vi "acquireValue.vi"(8 "error in (no error)":errorcluster, 10 "nextSample?":bool, 11 "appliedSettingsMatchStart in":refnum<class "appliedSettingsMatchStart.lvclass">) -> (0 "error out":errorcluster, 1 "function return":i32, 2 "variantData":variant, 3 "appliedSettingsMatchStart out":refnum<class "appliedSettingsMatchStart.lvclass">)   [LabVIEW 2016, in "SALLV_AtDome_Messaging.lvlib" / "appliedSettingsMatchStart.lvclass"]
uses:
  appliedSettingsMatchStart.lvclass
  appliedSettingsMatchStart.lvclass/appliedSettingsMatchStart.ctl
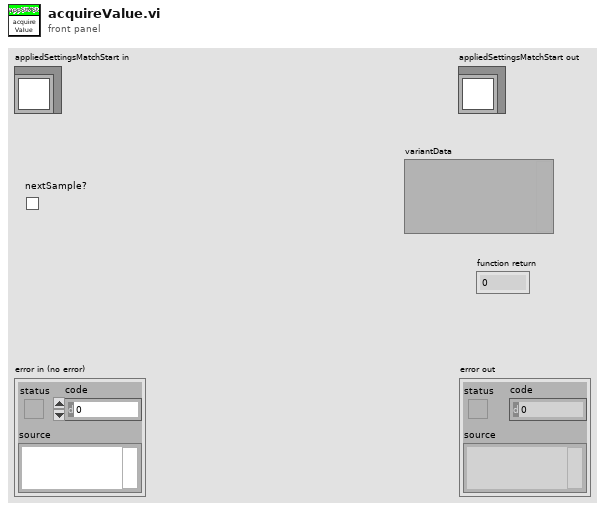
[diagram p1: front panel]
types:
  T1 = typedef "SALLV_EXA.lvlib/logevent_appliedSettingsMatchStart.ctl" = cluster{"appliedSettingsMatchStartIsTrue":bool, "priority":i32}
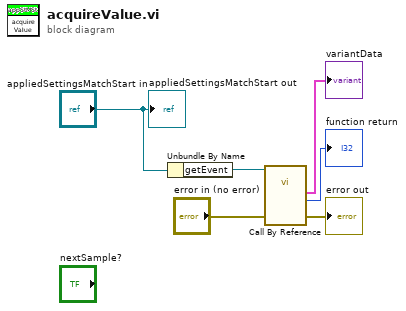
[diagram p0: block diagram]
diagram:
  n1 = Unbundle By Name("appliedSettingsMatchStart in") -> ("getEvent"=w6:refnum<vi>)
  n2 = call-by-ref "?"(reference=w6, "error in (no error)"="error in (no error)") -> ("error out"=→"error out":errorcluster, "function return"=→"function return":i32, "logevent_appliedSettingsMatchStart_Ctl out"=→"variantData":T1)  [unwired: 9 in, 2 out]
  "appliedSettingsMatchStart out" <- "appliedSettingsMatchStart in"
